vi "RichToFlatnixnet_grpc_ReadSignalWaveformResponse.vi"(5 "OutputClusterType":T1, 11 "InputCluster":T2) -> (3 "OutputCluster":T1)   [LabVIEW 2025, in "xnet-grpc_client.lvlib"]
uses:
  nixnet_grpc_ReadSignalWaveformResponse.ctl
  nixnet_grpc_ReadSignalWaveformResponse_Flat.ctl
  xnet-grpc_client.lvlib
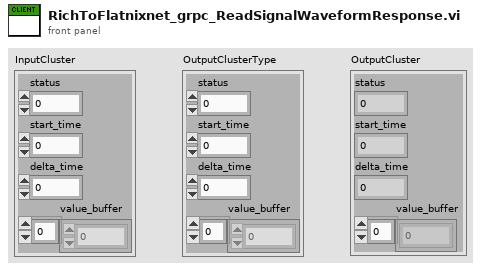
[diagram p1: front panel]
types:
  T1 = typedef "xnet-grpc_client.lvlib/nixnet_grpc_ReadSignalWaveformResponse_Flat.ctl" = cluster{"status":i32, "start_time":u64, "delta_time":dbl, "value_buffer":dbl[]}
  T2 = typedef "xnet-grpc_client.lvlib/nixnet_grpc_ReadSignalWaveformResponse.ctl" = cluster{"status":i32, "start_time":u64, "delta_time":dbl, "value_buffer":dbl[]}
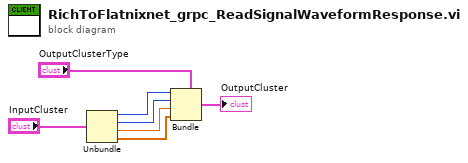
[diagram p0: block diagram]
diagram:
  n1 = Unbundle "Unbundle"("InputCluster") -> ("status"=w4:i32, "start_time"=w3:u64, "delta_time"=w2:dbl, "value_buffer"=w1:dbl[])
  n2 = Bundle "Bundle"(cluster="OutputClusterType", "status"=w4, "start_time"=w3, "delta_time"=w2, "value_buffer"=w1) -> (→"OutputCluster":T1)
